vi "AppConfigXMLToType.vi"(8 "error in (no error)":errorcluster, 10 "Config in":variant, 11 "RingdownPlugin in":refnum<class "EraPlugin.lvclass">) -> (0 "error out":errorcluster, 3 "RingdownPlugin out":refnum<class "EraPlugin.lvclass">)   [LabVIEW 2017, in "AppPlugins.lvlib" / "ERAPlugin.lvclass"]
uses:
  EraPlugin.lvclass
  PublicAPI/TypeDef/RingdownConfig.ctl
  EraPlugin.lvclass/EraPlugin.ctl
  Accessors/Write RingdownConfig.vi
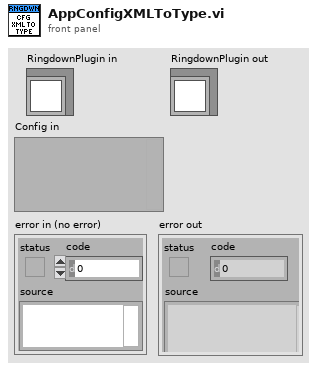
[diagram p1: front panel]
types:
  T1 = typedef "AppPlugins.lvlib/ERAPlugin.lvclass/RingdownConfig.ctl" = cluster{"Config":cluster{"p_SysOdr":i32, "dThres":dbl, "Preproc":cluster{"order":i32, "f_lo":dbl, "f_hi":dbl, "R_down":i32}}, "V index":i32, "I index":i32, "PosSeq":bool}
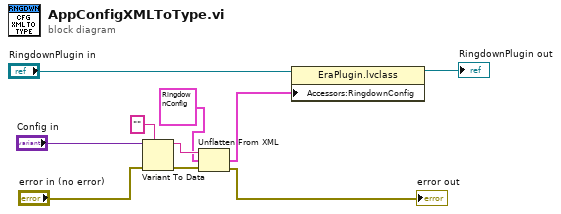
[diagram p0: block diagram]
diagram:
  n1 = Variant To Data(error in="error in (no error)", type="", Variant="Config in") -> (data=w7:string, error out=w6:errorcluster)
  n2 = Unflatten From XML(xml string=w7, type=T1 {"Config"={"p_SysOdr"=-1, "dThres"=0.0, "Preproc"={"order"=0, "f_lo"=1000.0, "f_hi"=1000.0, "R_down"=-1}}, "V index"=0, "I index"=3, "PosSeq"=FALSE} ("RingdownConfig"), error in (no error)=w6) -> (value=w1:T1, error out=→"error out":errorcluster)
  n3 = property class="EraPlugin.lvclass"(reference="RingdownPlugin in", "Accessors:RingdownConfig"=w1) -> (reference out=→"RingdownPlugin out":refnum<class "EraPlugin.lvclass">)  [unwired: 1 in, 1 out]
